vi "SSC Relay Control Multiple Actions.vi"(0 "SSC Relay in":T1[](array[typedef]), 5 "Relay Actions":T3[](array[typedef]) items=["Open Relay"=20, "Close Relay"=21], 7 "Settling Time (s)":dbl, 11 "error in":errorcluster) -> (4 "SSC Relay out":T1[](array[typedef]), 8 "Completed Relay Operations":T2[](array[typedef]) {"Desired State" items=["Open Relay"=20, "Close Relay"=21]}, 15 "error out":errorcluster)   [LabVIEW 2019]
doc: "Performs the specified relay actions on the Relays configured in the SSC Relay session. The function will then wait a specified amount of time if the Settling Time (s) input is wired. \n\nThere must be at exactly one Relay Action per Relay configured in the SSC Relay session, otherwise the function will return an error."
uses:
  <instrlib>/niSwitch/niSwitch.llb/niSwitch Relay Action.ctl
  SSC Relay.ctl
  SubVIs/TSM Relay Completed Operations.ctl
  Single SSC Relay NI-Switch Control.vi
  Single SSC Relay Fill Additional Error info.vi
  SSC Relay Expand Action Array to All Sessions.vi
  <instrlib>/niSwitch/niSwitch.llb/niSwitch Get Relay Position.vi
  <instrlib>/niSwitch/niSwitch.llb/niSwitch Relay Control.vi
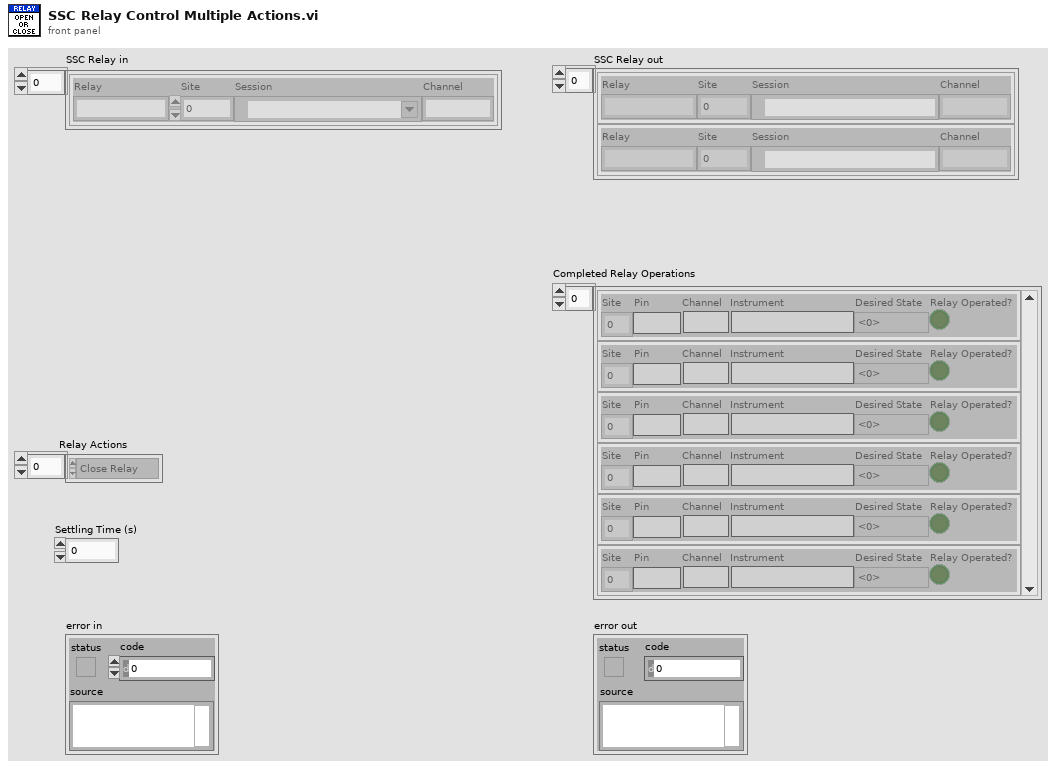
[diagram p1: front panel]
types:
  T1 = typedef "SSC Relay.ctl" = cluster{"Relay":string, "Site":i32, "Session":refnum<k15>, "Channel":string}
  T2 = typedef "TSM Relay Completed Operations.ctl" = cluster{"Site":i32, "Pin":string, "Channel":string, "Instrument":string, "Desired State":T3, "Relay Operated?":bool}
  T3 = typedef "niSwitch Relay Action.ctl" = i32
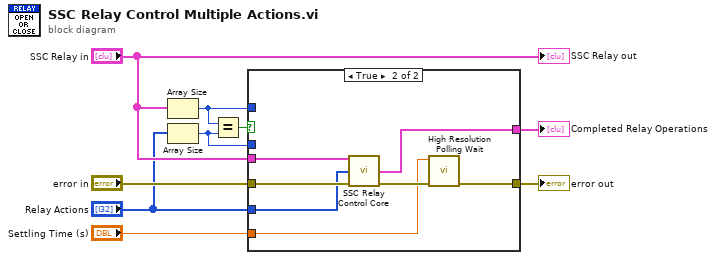
[diagram p0: block diagram]
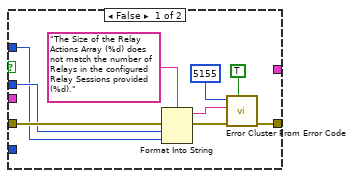
[diagram p2: hidden frame]
diagram:
  n1 = Array Size(array="SSC Relay in") -> (size(s)=w9:i32)
  n2 = Array Size(array="Relay Actions") -> (size(s)=w8:i32)
  n3 = Equal?(x=w9, y=w8) -> (x = y?=w1:bool)
  n4 = case shown="True" w1 {
    tunnel: [w15 w25] -> w5
    tunnel: "error in" -> [w16 w24]
    tunnel: [_ w21] -> w4
    tunnel: "Settling Time (s)" -> [_ w19]
    tunnel: "SSC Relay in" -> [_ w22]
    tunnel: "Relay Actions" -> [_ w20]
    tunnel: w9 -> [w10 _]
    tunnel: w8 -> [w11 _]
    frame False {
      n5 = Format Into String(format string="The Size of the Relay Actions Array (%d) does not match the number of Relays in the configured Relay Sessions provided (%d)." ("error message (\"\")"), error in=w16, w11, w10) -> (resulting string=w12:string, error out=w14:errorcluster)  [unwired: 1 in]
      n6 = call <vilib>:"Error Cluster From Error Code.vi"("show call chain? (False)"=TRUE, "error in (no error)"=w14, "error message (\"\")"=w12, "error code (0)"=5155) -> ("error out"=w15:errorcluster)  [unwired: 5 in]
    }
    frame True {
      n7 = call "SSC Relay Control Core.vi"("SSC Relay in"=w22, "Relay Commands"=w20, "error in"=w24) -> ("Completed Relay Operations"=w21:T2[], "error out"=w23:errorcluster)  [unwired: 10 in, 1 out]
      n8 = call <vilib>:"High Resolution Polling Wait.vi"("error in (no error)"=w23, "seconds to wait"=w19) -> ("error out"=w25:errorcluster)  [unwired: 9 in]
    }
  }
  "error out" <- w5
  "Completed Relay Operations" <- w4
  "SSC Relay out" <- "SSC Relay in"
